vi "Metric To Prometheus Lines.vi"(8 "error in (no error)":errorcluster, 10 "Include Metadata":bool=TRUE, 11 "Metrics.lvlib:Metric.lvclass":refnum<class "Metric.lvclass">) -> (0 "error out":errorcluster, 3 "Prometheus Lines":string[](array[string]))   [LabVIEW 2020, in "Metrics.lvlib" / "Metric.lvclass"]
uses:
  Metric.lvclass
  Metric.lvclass/Metric.ctl
  Read Name.vi
  Read Samples.vi
  Read Description.vi
  sample/Sample.lvclass
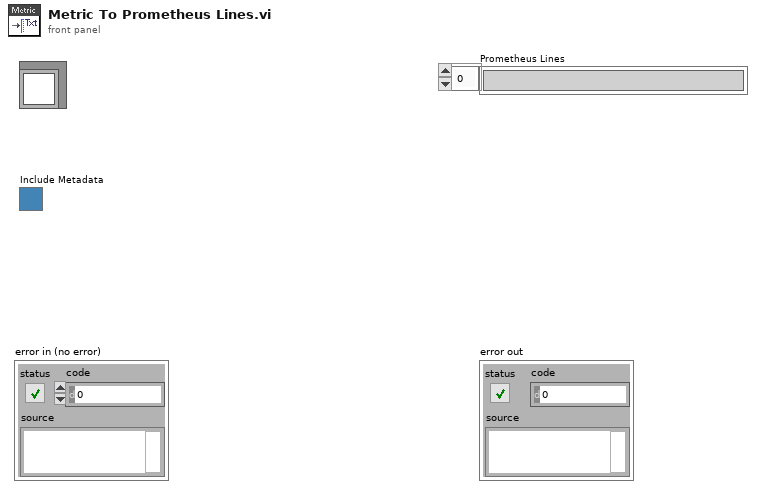
[diagram p1: front panel]
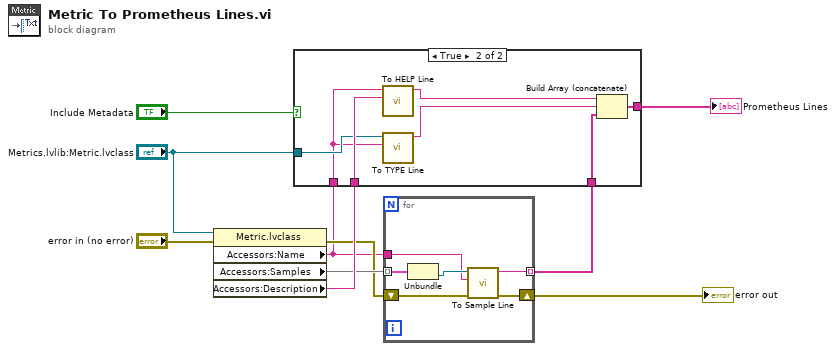
[diagram p0: block diagram]
diagram:
  n1 = property class="Metric.lvclass"(reference="Metrics.lvlib:Metric.lvclass", error in="error in (no error)") -> (error out=w5:errorcluster, "Accessors:Name"=w3:string, "Accessors:Samples"=w7:map{string, refnum<class "Sample.lvclass">}, "Accessors:Description"=w8:string)  [unwired: 1 out]
  n2 = for {
    tunnel: w7 -> [w13] mode=indexing
    tunnel: [w16] -> w9 mode=indexing
    shift-right: [w14] -> w1
    shift-left: w5 -> [w15]
    tunnel: w3 -> [w11]
    n3 = Unbundle(w13) -> (w12:refnum<class "Sample.lvclass">)  [unwired: 1 out]
    n4 = call "To Sample Line.vi"("error in (no error)"=w15, "Metric Name"=w11, "Sample in"=w12) -> ("error out"=w14:errorcluster, "Sample line"=w16:string)  [unwired: 7 in]
  }
  "error out" <- w1
  n5 = case shown="True" "Include Metadata" {
    tunnel: [w17 w24] -> w10
    tunnel: w9 -> [w17 w23]
    tunnel: w8 -> [_ w22]
    tunnel: "Metrics.lvlib:Metric.lvclass" -> [_ w21]
    tunnel: w3 -> [_ w20]
    frame False {
    }
    frame True {
      n6 = call "To HELP Line.vi"("Description"=w22, "Name"=w20) -> ("HELP line"=w18:string)  [unwired: 8 in, 1 out]
      n7 = call "To TYPE Line.vi"("Name"=w20, "Metric"=w21) -> ("TYPE line"=w19:string)  [unwired: 8 in, 1 out]
      n8 = Build Array (concatenate)(w18, w19, w23) -> (w24:string[])
    }
  }
  "Prometheus Lines" <- w10
